vi "PH_SHS_Analysis.PC Write PSDB.vi"(0 "i ref in":refnum<vi>, 5 "error IO":errorcluster) -> (14 "i ref out":refnum<vi>, 19 "error out":errorcluster)   [LabVIEW 2014, in "PH_SHS_Analysis.lvlib"]
doc: "This is the proc case which sets the data to be written to the to the PHELIX shot data base."
uses:
  PH_SHS_Analysis.lvlib
  PH_Basics/PH_PSDBWriter/PH_PSDBWriter.lvlib
  PH_Basics/PH_Img_BaseClass/PH_Img_BaseClass.lvlib
  PH_Basics/PH_StatusHandler/PH_StatusHandler.lvlib
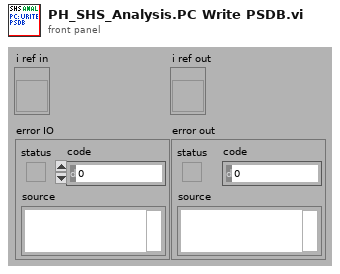
[diagram p1: front panel]
types:
  T1 = typedef "PH_SHS_Analysis.lvlib/PH_SHS_Analysis.i attribute.ctl" = cluster{"GUI Refs":cluster{"Delete":refnum<vi>, "Global On":refnum<vi>, "Cam Source":refnum<vi>, "Calibration Data File":refnum<vi>, "Calibration status":refnum<vi>, "Show overlay":refnum<vi>, "SHS Device Config":refnum<vi>, "Result":refnum<vi>, "Consider Tilt":refnum<vi>, "Working Reference":refnum<vi>, "Remove Tilt":refnum<vi>, "Take Cali  Reference":refnum<vi>, "Publishing Data Status":refnum<vi>, "Calibration Data":refnum<vi>}, "Calibration":cluster{"Status":T2, "Data":T3, "File":path}, "Result":T8, "Image":T11, "SHS Device Config":T12, "Show Overlay":bool, "GradientZernikeMatrix":dbl[][], "Consider Tilt":bool, "Working Reference":T4, "Zernicke Service ID":i32, "PSDB Image":T11}
  T2 = typedef "PH_StatusHandler.lvlib/PH_StatusHandler.Status.ctl" = i16
  T3 = typedef "PH_SHS_Analysis_Calibrator.lvlib/PH_SHS_Analysis_Calibrator.Analysis Calibration Data.ctl" = cluster{"Date":string, "Time":string, "Cam Settings":cluster{"Cam ID":string, "Gain":dbl, "Brightness":dbl, "Shutter":dbl, "Cam Error":bool, "Mode":i32}, "SHS Reference Result":T4, "Pixel Size":dbl, "MLA Pitch":dbl, "Method":enum16{"automatic", "manual"}, "Calibration Data calculated":bool, "No Problems at calculation?":bool, "error out":errorcluster}
  T4 = typedef "SHS_Common.lvlib/SHSReference.ctl" = cluster{"Reference":T5[][], "Lens Array Pitch [px]":dbl}
  T5 = typedef "SHS_Common.lvlib/ReferencePoint.ctl" = cluster{"Rect":T6, "Point":T7}
  T6 = typedef "SHS_Common.lvlib/Rectangle.ctl" = cluster{"Left":i32, "Top":i32, "Right":i32, "Bottom":i32}
  T7 = typedef "SHS_Common.lvlib/Point.ctl" = cluster{"x":dbl, "y":dbl, "valid?":bool, "weight":dbl}
  T8 = typedef "PH_SHS_Analysis.lvlib/PH_SHS_Analysis.Result.ctl" = cluster{"Time Stamp":timestamp, "Zernike Coefficients":T9, "PtV [lambda]":dbl, "Shifts":T10, "Measurement Quality":cluster{dbl, dbl, dbl}, "Measurement valid?":bool}
  T9 = typedef "PH_SHS_Analysis.lvlib/PH_SHS_Analysis.Zernike Coefficients.ctl" = cluster{"Tilt x":dbl, "Tilt y":dbl, "Defocus":dbl, "Astig 0°":dbl, "Astig 45°":dbl, "Coma x":dbl, "Coma y":dbl, "Spherical":dbl, "Trefoil 0°":dbl, "Trefoil 30°":dbl, "2nd Astig 0°":dbl, "2nd Astig 45°":dbl, "2nd Coma x":dbl, "2nd Coma y":dbl, "2nd Spherical":dbl}
  T10 = typedef "SHS_Common.lvlib/Shifts.ctl" = T7[][]
  T11 = typedef "IMAQ Image.ctl" = refnum<image>
  T12 = typedef "SHS_Analysis.lvlib/SHS_DeviceConfig.ctl" = cluster{"focal length [m]":dbl, "pixel size [m/px]":dbl, "wavelength [m]":dbl}
  T13 = typedef "PH_Img_BaseClass.lvlib/PH_Img_BaseClass.i attribute.ctl" = cluster{"GUI Refs":T14, "Timeout Image [ms]":i32, "Default Periodic Period [ms]":i32, "Camera":cluster{"Instancename":string, "Notifier":refnum<notifier>}, "Palette":T15, "Cam Settings":cluster{"Cam ID":string, "Gain":dbl, "Brightness":dbl, "Shutter":dbl, "Cam Info Failure":bool, "Mode":i32}}
  T14 = typedef "PH_Img_BaseClass.lvlib/PH_Img_BaseClass.GUI Refs.ctl" = cluster{"Timeout":refnum<vi>, "Image":refnum<vi>, "Palette":refnum<vi>, "Timeout Set":refnum<vi>}
  T15 = typedef "PH_Img_BaseClass.lvlib/PH_Img_BaseClass.Palette.ctl" = i32
  T16 = typedef "PH_PSDBWriter.lvlib/PH_PSDBWriter.String dataset.ctl" = cluster{"name":string, "data":string, "unit":string}
  T17 = typedef "PH_PSDBWriter.lvlib/PH_PSDBWriter.Numeric dataset.ctl" = cluster{"name":string, "data":dbl, "unit":string}
  T18 = typedef "PH_PSDBWriter.lvlib/PH_PSDBWriter.Image dataset.ctl" = cluster{"name":string, "data":T11, "unit":string}
  T19 = typedef "PH_PSDBWriter.lvlib/PH_PSDBWriter.PSDB Dataset.ctl" = cluster{"Version":i32, "2D data Input":T20[], "Boolean Input":T22[], "Image Input":T18[], "Numeric Input":T17[], "String Input":T16[]}
  T20 = typedef "PH_PSDBWriter.lvlib/PH_PSDBWriter.2D dataset.ctl" = cluster{"name":string, "data":dbl[][], "axis description":T21}
  T21 = typedef "PSDB.lvlib/PSDB_AxisDescription.ctl" = cluster{"x axis label":string, "y axis label":string, "x axis unit":string, "y axis unit":string}
  T22 = typedef "PH_PSDBWriter.lvlib/PH_PSDBWriter.Boolean dataset.ctl" = cluster{"name":string, "data":bool, "unit":string}
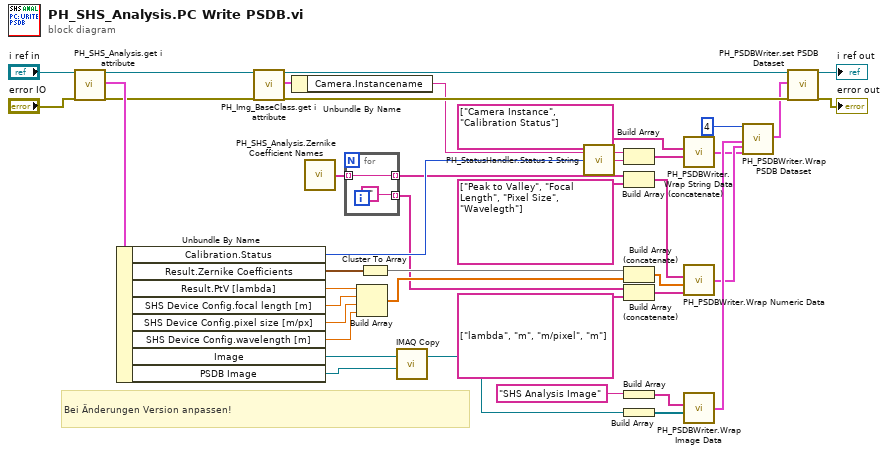
[diagram p0: block diagram]
diagram:
  # "Bei Änderungen Version anpassen!"
  n1 = call "PH_SHS_Analysis.get i attribute.vi"("i ref in"="i ref in", "error in (no error)"="error IO") -> ("i ref out"=w36:refnum<vi>, "i attribute"=w38:T1, "error out"=w20:errorcluster)  [unwired: 15 in]
  n2 = Unbundle By Name(w38) -> ("Calibration.Status"=w34:T2, "Result.Zernike Coefficients"=w32:T9, "Result.PtV [lambda]"=w28:dbl, "SHS Device Config.focal length [m]"=w27:dbl, "SHS Device Config.pixel size [m/px]"=w26:dbl, "SHS Device Config.wavelength [m]"=w25:dbl, "Image"=w3:T11, "PSDB Image"=w2:T11)
  n3 = call "PH_Img_BaseClass.get i attribute.vi"("i ref in"=w36, "error in (no error)"=w20) -> ("i ref out"=w18:refnum<vi>, "i attribute"=w33:T13, "error out"=w37:errorcluster)  [unwired: 15 in]
  n4 = Unbundle By Name(w33) -> ("Camera.Instancename"=w1:string)
  n5 = call "PH_SHS_Analysis.Zernike Coefficient Names.vi"() -> ("Zernickes"=w21:string[])
  n6 = for {
    tunnel: [w42] -> w30 mode=indexing
    tunnel: [""] -> w22 mode=indexing
    tunnel: w21 -> [w42] mode=indexing
  }
  n7 = Build Array(w28, w27, w26, w25) -> (w24:dbl[])
  n8 = Cluster To Array(cluster=w32) -> (array=w31:dbl[])
  n9 = call "IMAQ Copy"("Image Dst"=w2, "Image Src"=w3) -> ("Image Dst Out"=w4:T11)  [unwired: 4 in, 1 out]
  n10 = call "PH_StatusHandler.Status 2 String.vi"("Status"=w34) -> ("Status as string"=w35:string)
  n11 = Build Array(w1, w35) -> (w11:string[])
  n12 = Build Array (concatenate)(w30, string[] ["Peak to Valley", "Focal Length", "Pixel Size", "Wavelegth"]) -> (w7:string[])
  n13 = Build Array (concatenate)(w31, w24) -> (w8:dbl[])
  n14 = Build Array (concatenate)(w22, string[] ["lambda", "m", "m/pixel", "m"]) -> (w9:string[])
  n15 = Build Array("SHS Analysis Image") -> (w5:string[])
  n16 = Build Array(w4) -> (w6:T11[])
  n17 = call "PH_PSDBWriter.Wrap String Data.vi"("Data Array"=w11, "Name Array"=string[] ["Camera Instance", "Calibration Status"]) -> ("PSDB String Data Array"=w13:T16[])  [unwired: 2 in]
  n18 = call "PH_PSDBWriter.Wrap Numeric Data.vi"("Unit Array"=w9, "Data Array"=w8, "Name Array"=w7) -> ("PSDB Numeric Data Array"=w14:T17[])  [unwired: 1 in]
  n19 = call "PH_PSDBWriter.Wrap Image Data.vi"("Data Arrray"=w6, "Name Array"=w5) -> ("PSDB Image Data Array"=w15:T18[])  [unwired: 2 in]
  n20 = call "PH_PSDBWriter.Wrap PSDB Dataset.vi"("Version"=4, "Image Input"=w15, "Numeric Input"=w14, "String Input"=w13) -> ("PSDB Dataset"=w16:T19)  [unwired: 15 in]
  n21 = call "PH_PSDBWriter.set PSDB Dataset.vi"("VI in"=w18, "PSDB Dataset"=w16, "error in (no error)"=w37) -> ("VI out"=→"i ref out":refnum<vi>, "error out"=→"error out":errorcluster)  [unwired: 15 in]
